vi "getImages.vi"(6 "Settings.number of cam":dbl, 10 "data":T1, 11 "SubscriberCluster":T3) -> (0 "B[mT]":dbl, 1 "Images":T5, 2 "ROI":T6, 3 "OK":bool[](array[boolean]), 4 "Numeric":u32, 5 "Y size":i32[](array[numeric]))   [LabVIEW 2011, in "MagAnalysis_Online.lvclass"]
uses:
  MagAnalysis_Online.lvclass
  ROIStartfromCam_typdef.ctl
  analysis_data_typdef.ctl
  IMAQ Image.ctl
  dataTypdef.ctl
  SubscriberCluster_TypDEf.ctl
  tcp_new_data_event.ctl
  tcp new data cluster.ctl
panel:
  out "data 2":T1
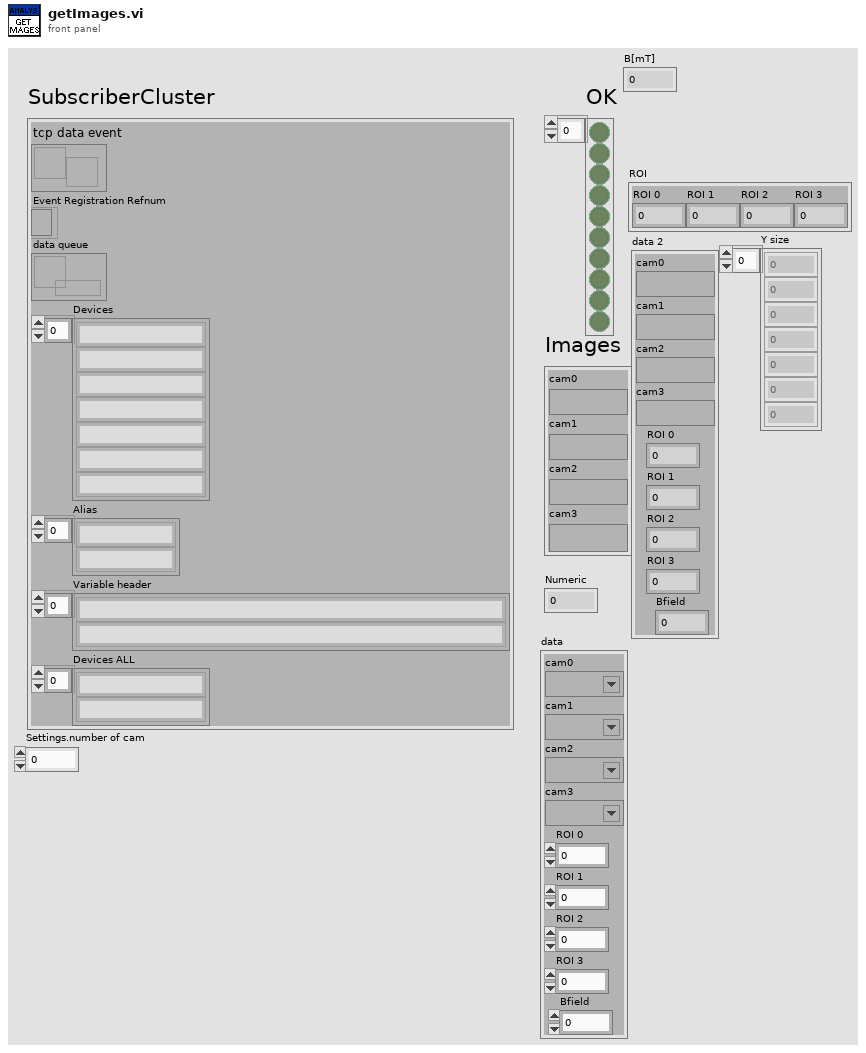
[diagram p1: front panel]
types:
  T1 = typedef "dataTypdef.ctl" = cluster{"cam0":T2, "cam1":T2, "cam2":T2, "cam3":T2, "ROI 0":dbl, "ROI 1":dbl, "ROI 2":dbl, "ROI 3":dbl, "Bfield":dbl}
  T2 = typedef "IMAQ Image.ctl" = refnum<image>
  T3 = typedef "SubscriberCluster_TypDEf.ctl" = cluster{"tcp data event":T4, "Event Registration Refnum":refnum<event-registration>, "data queue":refnum<queue>, "Devices":string[], "Alias":string[], "Variable header":string[], "Devices ALL":string[]}
  T4 = typedef "tcp_new_data_event.ctl" = refnum<user-event>
  T5 = typedef "MagAnalysis_Online.lvclass/analysis_data_typdef.ctl" = cluster{"cam0":T2, "cam1":T2, "cam2":T2, "cam3":T2}
  T6 = typedef "ROIStartfromCam_typdef.ctl" = cluster{"ROI 0":dbl, "ROI 1":dbl, "ROI 2":dbl, "ROI 3":dbl}
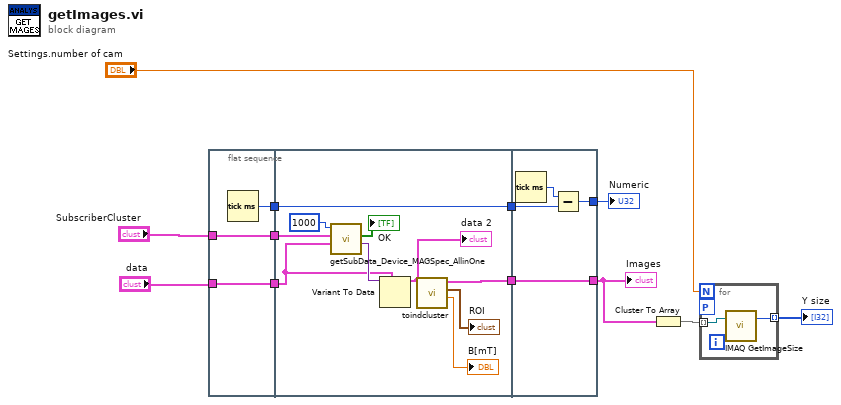
[diagram p0: block diagram]
diagram:
  n1 = flat-sequence {
    tunnel: "data" -> [w14]
    tunnel: "SubscriberCluster" -> [w15]
    tunnel: [w15] -> w12
    tunnel: [w14] -> w11
    tunnel: [w13] -> w10
    tunnel: [w20] -> w9
    tunnel: w12 -> [w25]
    tunnel: w11 -> [w22]
    tunnel: w10 -> [w18]
    tunnel: [w18] -> w8
    tunnel: [w29] -> w5
    tunnel: w9 -> [w29]
    tunnel: w8 -> [w27]
    tunnel: [w26] -> w7
    frame #0 {
      n2 = Tick Count (ms)() -> (millisecond timer value=w13:u32)
    }
    frame #1 {
      n3 = call "getSubData_Device_MAGSpec_AllinOne.vi"("variant in"=w22, "SubscriberCluster"=w25, "timeout"=1000) -> ("variant out"=w23:variant, "OK"=→"OK":bool[])  [unwired: 7 in]
      n4 = Variant To Data(type=w22, Variant=w23) -> (data=w16:T1)  [unwired: 1 in, 1 out]
      "data 2" <- w16
      n5 = call "toindcluster.vi"("data"=w16) -> ("B[mT]"=→"B[mT]":dbl, "ROI"=→"ROI":T6, "Images"=w20:T5)  [unwired: 8 in]
    }
    frame #2 {
      n6 = Tick Count (ms)() -> (millisecond timer value=w28:u32)
      n7 = Subtract(x=w28, y=w27) -> (x-y=w26:u32)
    }
  }
  n8 = Cluster To Array(cluster=w5) -> (array=w4:T2[])
  n9 = for {
    N: "Settings.number of cam" -> [_]
    tunnel: w4 -> [w31] mode=indexing
    workers-P: _ -> [_]
    tunnel: [w30] -> w3 mode=indexing
    n10 = call "IMAQ GetImageSize"("Image"=w31) -> ("Y Resolution"=w30:i32)  [unwired: 3 in, 2 out]
  }
  "Y size" <- w3
  "Numeric" <- w7
  "Images" <- w5
